vi "FT10_M4X Set Parameter.vi"(8 "error in (no error)":errorcluster, 9 "Value":i32, 10 "Register":i32, 11 "Card Handle in":u32) -> (0 "error out":errorcluster, 3 "Card Handle out":u32)   [LabVIEW 2024]
doc: "Copy of \"M4X_Set_Parameter.vi\" from HWT_Lillis_7854.lvproj"
uses:
  LV2015/Transfer dlls/spcm_win32.dll
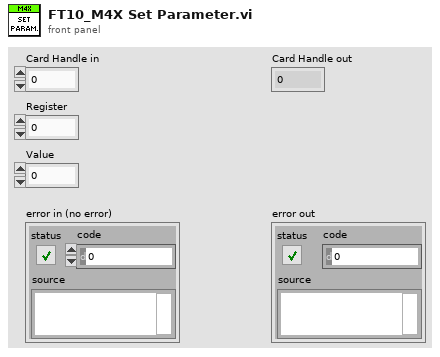
[diagram p1: front panel]
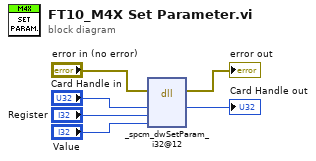
[diagram p0: block diagram]
diagram:
  n1 = dll-call lib="C:/Users/yearon2/OneDrive - Medtronic PLC/LV2015/Transfer dlls/spcm_win32.dll" fn="_spcm_dwSetParam_i32@12"(error in="error in (no error)", "hDrv"="Card Handle in", "lRegister"="Register", "lValue"="Value") -> (error out=→"error out":errorcluster, "hDrv"=→"Card Handle out":u32)  [unwired: 5 in, 1 out]
